vi "host.vi"() -> ()   [LabVIEW 2018]
uses:
  <vilib>/userdefined/High Color/nirio_resource_hc.ctl
  <instrlib>/niDCPower/nidcpower.llb/niDCPower Measurement Type.ctl
  <vilib>/FPGAPlugInAG/PXI-7953R/niLvFpga_Open_PXI-7953R.vi
  <vilib>/rvi/interface/common/dynamic/niFpgaDynamicAddResources.vi
  <vilib>/FPGAPlugInAG/Dynamic/niLvFpga_Reset_Dynamic.vi
  <vilib>/FPGAPlugInAG/Dynamic/niLvFpga_Run_Dynamic.vi
  <vilib>/Utility/error.llb/Error Cluster From Error Code.vi
  <vilib>/rvi/errors/niLvFpgaAdjustHostInterfaceError.vi
  <vilib>/FPGAPlugInAG/Dynamic/niLvFpga_Close_Dynamic.vi
  <vilib>/rvi/interface/nirviOpenFPGA/nirviOpenFPGA.xnode
  FPGA Bitfiles/matrix_FPGATarget_Matrixtarget_8M6uhoGy8lc.lvbitx
  <vilib>/rvi/interface/nirviMethod/nirviMethod.xnode
  <vilib>/rvi/interface/nirviReadWriteControl/nirviReadWriteControl.xnode
  <vilib>/rvi/interface/nirviCloseFPGA/nirviCloseFPGA.xnode
  <vilib>/FPGAPlugInAG/Dynamic/niLvFpga_ReadFifo_Dynamic.vi
  <vilib>/rvi/errors/niLvFpgaMergeErrorWithErrorCode.vi
  <vilib>/rvi/interface/Simulation/niFpgaSimulationCallBeginRW.vi
  <vilib>/vision/NI_Vision_Development_Module.lvlib
  NiFpgaLv.dll
panel:
  out "glitch_sum":i32=137
  in  "INIT_REGISTERS":bool
  out "Glitch Report":string="--Report-- 1\r\np0#R9 rd 29F  df  00219 \r\n--Report-- 1\r\np0#R9 rd 29F  df  00219 \r\n--Report-- 0\r\n\r\n--Report-- 0\r\n\r\n--Report-- 1\r\np1#R146 rd FF  df  BF1E \r\n--Report-- 0\r\n\r\n--Report-- 0\r\n\r\n--Report-- 0\r\n\r\n--Report-- 0\r\n\r\n--Report-- 0\r\n\r\n--Report-- 3\r\np0#R4 rd 1E7  df  00500 p0#R9 rd 432  df  00219 p1#R58 rd 300  df  200 \r\n--Report-- 3\r\np0#R4 rd 1E7  df  00500 p0#R9 rd 432  df  00219 p1#R58 rd 300  df  200 \r\n--Report-- 3\r\np0#R4 rd 1E7  df  00500 p0#R9 rd 432  df  00219 p1#R58 rd 300  df  200 \r\n--Report-- 3\r\np0#R4 rd 1E7  df  00500 p0#R9 rd 432  df  00219 p1#R58 rd 300  df  200 \r\n--Report-- 3\r\np0#R4 rd 1E7  df  00500 p0#R9 rd 432  df  00219 p1#R58 rd 300  df  200 \r\n--Report-- 0\r\n\r\n--Report-- 1\r\np0#R9 rd 29F  df  00219 \r\n--Report-- 0\r\n\r\n--Report-- 137\r\np1#R155 rd 3  df  200 p1#R157 rd 3  df  24AE p1#R159 rd 3  df  0 p1#R160 rd 3  df  500 p1#R161 rd 3  df  500 p1#R162 rd 3  df  0 p1#R163 rd 3  df  400 p1#R164 rd 3  df  400 p1#R165 rd 3  df  0 p1#R166 rd 3  df  500 p1#R167 rd 3  df  280 p1#R168 rd 3  df  0 p1#R169 rd 3  df  400 p1#R170 rd 3  df  200 p1#R174 rd 3  df  504 p1#R175 rd 3  df  10 p1#R179 rd 3  df  2 p1#R180 rd 3  df  20 p1#R181 rd 3  df  101 p1#R182 rd 3  df  110B p1#R183 rd 3  df  3C27 p1#R184 rd 3  df  110A p1#R185 rd 3  df  3222 p1#R186 rd 3  df  160B p1#R187 rd 3  df  3224 p2#R2 rd 3  df  6E p2#R3 rd 3  df  2923 p2#R4 rd 3  df  524 p2#R9 rd 3  df  92 p2#R10 rd 3  df  16 p2#R11 rd 3  df  8 p2#R12 rd 3  df  AB p2#R13 rd 3  df  93 p2#R14 rd 3  df  58 p2#R15 rd 3  df  4D p2#R16 rd 3  df  A9 p2#R17 rd 3  df  A0 p2#R21 rd 3  df  175 p2#R22 rd 3  df  16 p2#R23 rd 3  df  43 p2#R24 rd 3  df  C p2#R25 rd 3  df  0 p2#R26 rd 3  df  15 p2#R27 rd 3  df  1F p2#R28 rd 3  df  16 p2#R29 rd 3  df  98 p2#R30 rd 3  df  4C p2#R31 rd 3  df  A0 p2#R32 rd 3  df  C814 p2#R33 rd 3  df  8080 p2#R34 rd 3  df  D960 p2#R35 rd 3  df  D960 p2#R36 rd 3  df  7F00 p2#R38 rd 3  df  8000 p2#R39 rd 3  df  8008 p2#R40 rd 3  df  EF04 p2#R41 rd 3  df  8D73 p2#R42 rd 3  df  D0 p2#R43 rd 3  df  6020 p2#R44 rd 3  df  6020 p2#R45 rd 3  df  F0A0 p2#R46 rd 3  df  C4A p2#R47 rd 3  df  DF20 p2#R51 rd 3  df  146E p2#R54 rd 3  df  7810 p2#R55 rd 3  df  300 p2#R56 rd 3  df  440 p2#R57 rd 3  df  68C p2#R58 rd 3  df  68C p2#R59 rd 3  df  68C p2#R60 rd 3  df  68C p2#R61 rd 3  df  17D9 p2#R62 rd 3  df  1CFF p2#R70 rd 3  df  D900 p2#R87 rd 3  df  219 p2#R88 rd 3  df  284 p2#R89 rd 3  df  219 p2#R90 rd 3  df  284 p2#R92 rd 3  df  120C p2#R93 rd 3  df  1512 p2#R94 rd 3  df  683C p2#R95 rd 3  df  3008 p2#R96 rd 3  df  2 p2#R100 rd 3  df  59FC p2#R101 rd 3  df  0 p2#R103 rd 3  df  4010 p2#R104 rd 3  df  11 p2#R130 rd 3  df  3FC p2#R131 rd 3  df  301 p2#R132 rd 3  df  C1 p2#R133 rd 3  df  3A1 p2#R134 rd 3  df  3D4 p2#R135 rd 3  df  3D7 p2#R136 rd 3  df  399 p2#R137 rd 3  df  3F8 p2#R138 rd 3  df  1C p2#R139 rd 3  df  3BD p2#R140 rd 3  df  3DB p2#R141 rd 3  df  3BD p2#R142 rd 3  df  3FC p2#R143 rd 3  df  3DE p2#R144 rd 3  df  3DE p2#R145 rd 3  df  3DE p2#R146 rd 3  df  3DE p2#R147 rd 3  df  1F p2#R148 rd 3  df  41 p2#R149 rd 3  df  363 p2#R150 rd 3  df  0 p2#R152 rd 3  df  FF p2#R153 rd 3  df  1 p2#R156 rd 3  df  DF20 p2#R180 rd 3  df  20 p2#R198 rd 3  df  0 p2#R200 rd 3  df  0 p2#R203 rd 3  df  0 p2#R204 rd 3  df  0 p2#R205 rd 3  df  21A0 p2#R206 rd 3  df  1E9B p2#R207 rd 3  df  4A4A p2#R208 rd 3  df  168D p2#R209 rd 3  df  4D p2#R210 rd 3  df  0 p2#R211 rd 3  df  0 p2#R212 rd 3  df  208 p2#R213 rd 3  df  0 p2#R239 rd 3  df  8 p2#R242 rd 3  df  0 p2#R244 rd 3  df  6E p2#R246 rd 3  df  36 p2#R247 rd 3  df  D p2#R248 rd 3  df  AB p2#R249 rd 3  df  88 p2#R250 rd 3  df  48 p2#R251 rd 3  df  57 p2#R252 rd 3  df  5E p2#R253 rd 3  df  7A p2#R254 rd 3  df  503F \r\n"
  in  "REGISTERS":bool=TRUE
  in  "GLITCH":path=path "C:/TIM/Project/Matrix/Logs/Control/GLITCH"
  out "GLITCH_log file":refnum<file>
  in  "Index - Registers Page 2":u16[](array[numeric])=[2, 3, 4, 9, 10, 11, 12, 13, 14, 15, 16, 17, 65535, 65535, 65535, 21, 22, 23, 24, 25, 26, 27, 28, 29, 30, 31, 32, 33, 34, 35, 36, 38, 39, 40, 41, 42, 43, 44, 45, 46, 47, 65535, 65535, 65535, 51, 54, 55, 56, 57, 58, 59, 60, 61, 62, 65535, 70, 65535, 65535, 65535, 65535, 87, 88, 89, 90, 65535, 92, 93, 94, 95, 96, 65535, 65535, 65535, 100, 101, 103, 104, 130, 131, 132, 133, 134, 135, 136, 137, 138, 139, 140, 141, 142, 143, 144, 145, 146, 147, 148, 149, 150, 152, 153, 156, 180, 198, 200, 203, 204, 205, 206, 207, 208, 209, 210, 211, 212, 213, 239, 65535, 242, 65535, 244, 246, 247, 248, 249, 250, 251, 252, 253, 254, 255, 65535, 65535, 65535, 65535, 65535, 65535, 65535, 65535, 65534, 65535, 65535, 65531, 241, 242, 243, 244, 245, 246, 247, 248, 249, 250, 251, 252, 253, 254, 255]
  in  "Registers Page 2":u16[](array[numeric])=[110, 10531, 1316, 146, 22, 8, 171, 147, 88, 77, 169, 160, 65535, 65535, 65535, 373, 22, 67, 12, 0, 21, 31, 22, 152, 76, 160, 51220, 32896, 55648, 55648, 32512, 32768, 32776, 61188, 36211, 208, 24608, 24608, 61600, 3146, 57120, 65535, 65535, 65535, 5230, 30736, 768, 1088, 1676, 1676, 1676, 1676, 6105, 7423, 65535, 55552, 0, 65535, 65535, 65535, 537, 644, 537, 644, 2, 4620, 5394, 26684, 12296, 2, 32896, 65535, 65535, 23036, 0, 16400, 17, 1020, 769, 193, 929, 980, 983, 921, 1016, 28, 957, 987, 957, 1020, 990, 990, 990, 990, 31, 65, 867, 0, 255, 1, 57120, 32, 0, 0, 0, 0, 8608, 7835, 19018, 5773, 77, 0, 0, 520, 0, 8, 0, 0, 0, 110, 54, 13, 171, 136, 72, 87, 94, 122, 20543, 43136] format="%x"
  in  "current limit VDDIO":dbl=0.1 format="%#_13g"
  in  "voltage level VDDIO":dbl=2.5 format="%#_13g"
  in  "57":i16=57
  in  "91":i16=91
  in  "Index - Registers Page 1":u16[](array[numeric])=[5, 6, 8, 16, 17, 18, 27, 28, 30, 37, 52, 53, 58, 59, 60, 71, 72, 76, 77, 78, 82, 83, 84, 85, 86, 87, 88, 104, 128, 129, 130, 131, 132, 133, 134, 135, 136, 137, 138, 139, 140, 141, 142, 143, 144, 145, 146, 147, 148, 149, 155, 157, 159, 160, 161, 162, 163, 164, 165, 166, 167, 168, 169, 170, 174, 175, 179, 180, 181, 182, 183, 184, 185, 186, 187, 188, 189, 190, 191, 192, 193, 194, 195, 196, 200, 220, 221, 222, 223, 224, 225, 226, 227, 240]
  in  "Registers Page 1":u16[](array[numeric])=[3, 28686, 128, 61437, 64831, 16367, 0, 0, 512, 5, 16, 61456, 512, 1066, 1024, 24, 0, 0, 0, 10, 0, 7700, 17966, 34666, 47008, 57548, 0, 17, 7, 56588, 62696, 1276, 57868, 63212, 764, 56588, 62696, 250, 34866, 56754, 63466, 2, 47646, 60627, 63473, 255, 48926, 61142, 63474, 3, 512, 9390, 0, 1280, 1280, 0, 1024, 1024, 0, 1280, 640, 0, 1024, 512, 1284, 16, 2, 32, 257, 4363, 15399, 4362, 12834, 5643, 12836, 9228, 24124, 127, 8200, 20023, 100, 8463, 19250, 100, 0, 7700, 17966, 34666, 47008, 57548, 0, 28672, 45091, 0] format="%x"
  out "Glitch Registers":string="p1#R155 rd 3  df  200 p1#R157 rd 3  df  24AE p1#R159 rd 3  df  0 p1#R160 rd 3  df  500 p1#R161 rd 3  df  500 p1#R162 rd 3  df  0 p1#R163 rd 3  df  400 p1#R164 rd 3  df  400 p1#R165 rd 3  df  0 p1#R166 rd 3  df  500 p1#R167 rd 3  df  280 p1#R168 rd 3  df  0 p1#R169 rd 3  df  400 p1#R170 rd 3  df  200 p1#R174 rd 3  df  504 p1#R175 rd 3  df  10 p1#R179 rd 3  df  2 p1#R180 rd 3  df  20 p1#R181 rd 3  df  101 p1#R182 rd 3  df  110B p1#R183 rd 3  df  3C27 p1#R184 rd 3  df  110A p1#R185 rd 3  df  3222 p1#R186 rd 3  df  160B p1#R187 rd 3  df  3224 p2#R2 rd 3  df  6E p2#R3 rd 3  df  2923 p2#R4 rd 3  df  524 p2#R9 rd 3  df  92 p2#R10 rd 3  df  16 p2#R11 rd 3  df  8 p2#R12 rd 3  df  AB p2#R13 rd 3  df  93 p2#R14 rd 3  df  58 p2#R15 rd 3  df  4D p2#R16 rd 3  df  A9 p2#R17 rd 3  df  A0 p2#R21 rd 3  df  175 p2#R22 rd 3  df  16 p2#R23 rd 3  df  43 p2#R24 rd 3  df  C p2#R25 rd 3  df  0 p2#R26 rd 3  df  15 p2#R27 rd 3  df  1F p2#R28 rd 3  df  16 p2#R29 rd 3  df  98 p2#R30 rd 3  df  4C p2#R31 rd 3  df  A0 p2#R32 rd 3  df  C814 p2#R33 rd 3  df  8080 p2#R34 rd 3  df  D960 p2#R35 rd 3  df  D960 p2#R36 rd 3  df  7F00 p2#R38 rd 3  df  8000 p2#R39 rd 3  df  8008 p2#R40 rd 3  df  EF04 p2#R41 rd 3  df  8D73 p2#R42 rd 3  df  D0 p2#R43 rd 3  df  6020 p2#R44 rd 3  df  6020 p2#R45 rd 3  df  F0A0 p2#R46 rd 3  df  C4A p2#R47 rd 3  df  DF20 p2#R51 rd 3  df  146E p2#R54 rd 3  df  7810 p2#R55 rd 3  df  300 p2#R56 rd 3  df  440 p2#R57 rd 3  df  68C p2#R58 rd 3  df  68C p2#R59 rd 3  df  68C p2#R60 rd 3  df  68C p2#R61 rd 3  df  17D9 p2#R62 rd 3  df  1CFF p2#R70 rd 3  df  D900 p2#R87 rd 3  df  219 p2#R88 rd 3  df  284 p2#R89 rd 3  df  219 p2#R90 rd 3  df  284 p2#R92 rd 3  df  120C p2#R93 rd 3  df  1512 p2#R94 rd 3  df  683C p2#R95 rd 3  df  3008 p2#R96 rd 3  df  2 p2#R100 rd 3  df  59FC p2#R101 rd 3  df  0 p2#R103 rd 3  df  4010 p2#R104 rd 3  df  11 p2#R130 rd 3  df  3FC p2#R131 rd 3  df  301 p2#R132 rd 3  df  C1 p2#R133 rd 3  df  3A1 p2#R134 rd 3  df  3D4 p2#R135 rd 3  df  3D7 p2#R136 rd 3  df  399 p2#R137 rd 3  df  3F8 p2#R138 rd 3  df  1C p2#R139 rd 3  df  3BD p2#R140 rd 3  df  3DB p2#R141 rd 3  df  3BD p2#R142 rd 3  df  3FC p2#R143 rd 3  df  3DE p2#R144 rd 3  df  3DE p2#R145 rd 3  df  3DE p2#R146 rd 3  df  3DE p2#R147 rd 3  df  1F p2#R148 rd 3  df  41 p2#R149 rd 3  df  363 p2#R150 rd 3  df  0 p2#R152 rd 3  df  FF p2#R153 rd 3  df  1 p2#R156 rd 3  df  DF20 p2#R180 rd 3  df  20 p2#R198 rd 3  df  0 p2#R200 rd 3  df  0 p2#R203 rd 3  df  0 p2#R204 rd 3  df  0 p2#R205 rd 3  df  21A0 p2#R206 rd 3  df  1E9B p2#R207 rd 3  df  4A4A p2#R208 rd 3  df  168D p2#R209 rd 3  df  4D p2#R210 rd 3  df  0 p2#R211 rd 3  df  0 p2#R212 rd 3  df  208 p2#R213 rd 3  df  0 p2#R239 rd 3  df  8 p2#R242 rd 3  df  0 p2#R244 rd 3  df  6E p2#R246 rd 3  df  36 p2#R247 rd 3  df  D p2#R248 rd 3  df  AB p2#R249 rd 3  df  88 p2#R250 rd 3  df  48 p2#R251 rd 3  df  57 p2#R252 rd 3  df  5E p2#R253 rd 3  df  7A p2#R254 rd 3  df  503F "
  out "glitch_num":i32=137
  out "Data_Read":u16=3 format="%x"
  in  "Index - Registers Page 0":u16[](array[numeric])=[0, 1, 2, 3, 4, 5, 6, 7, 8, 9, 10, 11, 12, 13, 31, 32, 33, 34, 35, 36, 65535, 65535, 65535, 65535, 65535, 48, 49, 50, 51, 52, 54, 55, 65535, 60, 61, 65535, 63, 64, 65, 66, 89, 90, 95, 96, 65535, 65535, 65535, 65535, 101, 112, 113, 114, 115, 116, 117, 118, 119, 120, 121, 122, 123, 124, 125, 126, 128, 129, 130, 131, 132, 133, 134, 135, 200, 240, 245, 246, 247, 248, 65535, 250, 251, 252, 253, 255, 65535]
  in  "Registers Page 0":u16[](array[numeric])=[5178, 12, 30, 1024, 1280, 388, 42, 190, 17, 537, 17, 0, 0, 8, 0, 768, 1036, 297, 1544, 32875, 32, 32, 32, 32, 32, 1066, 7168, 0, 841, 49177, 61680, 0, 33, 6688, 8222, 8224, 8224, 8220, 215, 1911, 12, 49167, 8989, 128, 0, 0, 0, 0, 0, 31498, 31498, 6414, 6159, 22322, 22068, 29493, 12306, 30978, 29958, 30474, 30729, 32006, 12560, 126, 127, 127, 22282, 22539, 18188, 18446, 23298, 92, 0, 0, 2047, 2047, 0, 0, 124, 0, 0, 0, 0, 5178] format="%x"
  out "number":u64=515396075521 format="%b"
  in  "WRITE\nSEL_LOG":bool=TRUE caption="SEL LOGS"
  out "SEL_log file":refnum<file>
  out "IS_SEL":bool
  in  "SIM_SEL":bool
  in  "VDDIO_limit, mA":dbl=20.0 format="%#_13g"
  in  "VAA_limit, mA":dbl=40.0 format="%#_13g"
  out "selNumVAA":i32 caption="selNum"
  out "selNumVDDIO":i32 caption="selNum"
  in  "voltage level VAA":dbl=2.8 format="%#_13g"
  in  "voltage level VDD":dbl=2.8 format="%#_13g"
  in  "current limit VAA":dbl=0.10000000000000009 format="%#_13g"
  in  "current limit VDD":dbl=0.1 format="%#_13g"
  in  "SEL":path=path "C:/TIM/Project/Matrix/Logs/Control/SEL"
  out "Температура":string="0"
  out "Номер образца":string="0"
  out "VDDIO_Current, mA":dbl=-0.05343834220867134 caption="mA" format="%_2g"
  out "VDDIO_Voltage, V":dbl=2.500600525204199 caption="V" format="%_3g"
  out "VAA_Current, mA":dbl=14.9087718833614 caption="mA" format="%_2g"
  out "VAA_Voltage, V":dbl=2.800387385516999 caption="V" format="%_3g"
  in  "VAA - VAAPIX":refnum<k15>="PXI1Slot2"
  in  "SEL_time":u32=100
  out "Read_Low":u8=3 format="%x"
  out "Read_Up":u8 format="%x"
  out "TIRISTOR":bool
  in  "/RESET":bool=TRUE
  in  "DataLow":u8=25 format="%x"
  in  "Reg":u8=254 format="%x"
  in  "DataUp":u8=2 format="%x"
  in  "Device":u8=186 format="%x"
  in  "VDD_limit, mA":dbl=20.0 format="%#_13g"
  out "selNumVDD":i32 caption="selNum"
  out "Ready":bool=TRUE
  in  "output enabled":bool=TRUE
  out "VDD_Current, mA":dbl=-0.3667932165298103 caption="mA" format="%_2g"
  out "VDD_Voltage, V":dbl=2.7994963728933535 caption="V" format="%_3g"
  in  "VDDIO - VDD":refnum<k15>="PXI1Slot3"
  in  "Comand":T1(ring)
  in  "Height_pix":i32=250
  in  "Width_pix":i32=250
  in  "55":i16=55
  in  "73":i16=73
  in  "75":i16=75
  in  "56":i16=56
  in  "55":i16=55
  in  "Comand":bool
  out "ACK":u8 format="%b"
  out "String_counter":i16=250
  in  "String_number":i16=250
  in  "I2C_Request":bool
  in  "FALSE_LV":bool
  in  "FALSE_PIXCLK":bool=TRUE
  in  "TRUE_FV":bool=TRUE
  in  "1_EXTCLK_divider":i16=1
  out "Image":T2(plugin-control)
  in  "0_WE divider":i32
  in  "50_Rise/Fall divider":i32=25
  in  "72":i16=72
  in  "18":i16=18
  in  "36":i16=36
  in  "54":i16=54
  in  "71":i16=71
  in  "17":i16=17
  in  "35":i16=35
  in  "53":i16=53
  in  "75_Stop":i16=75
  in  "100_Sclk_divider":i32=50
  in  "Read1":u8=255 format="%x"
  in  "Read2":u8=255 format="%x"
  in  "I2C_Write":bool
  in  "stop":bool=TRUE
  out "ArrayUp":u64=1432
  out "ArrayLow":u64=27021700977551334
  in  "resource name":T3="PXI1Slot6" caption="RIO Device"
  out "Сколько вначале":u32=262142
  out "Data":u8[](array[numeric])
  # "YCbCr mode"
  # "RGB565"
  # "VDD"
  # "VDDIO"
  # "VAA"
  # "I2C"
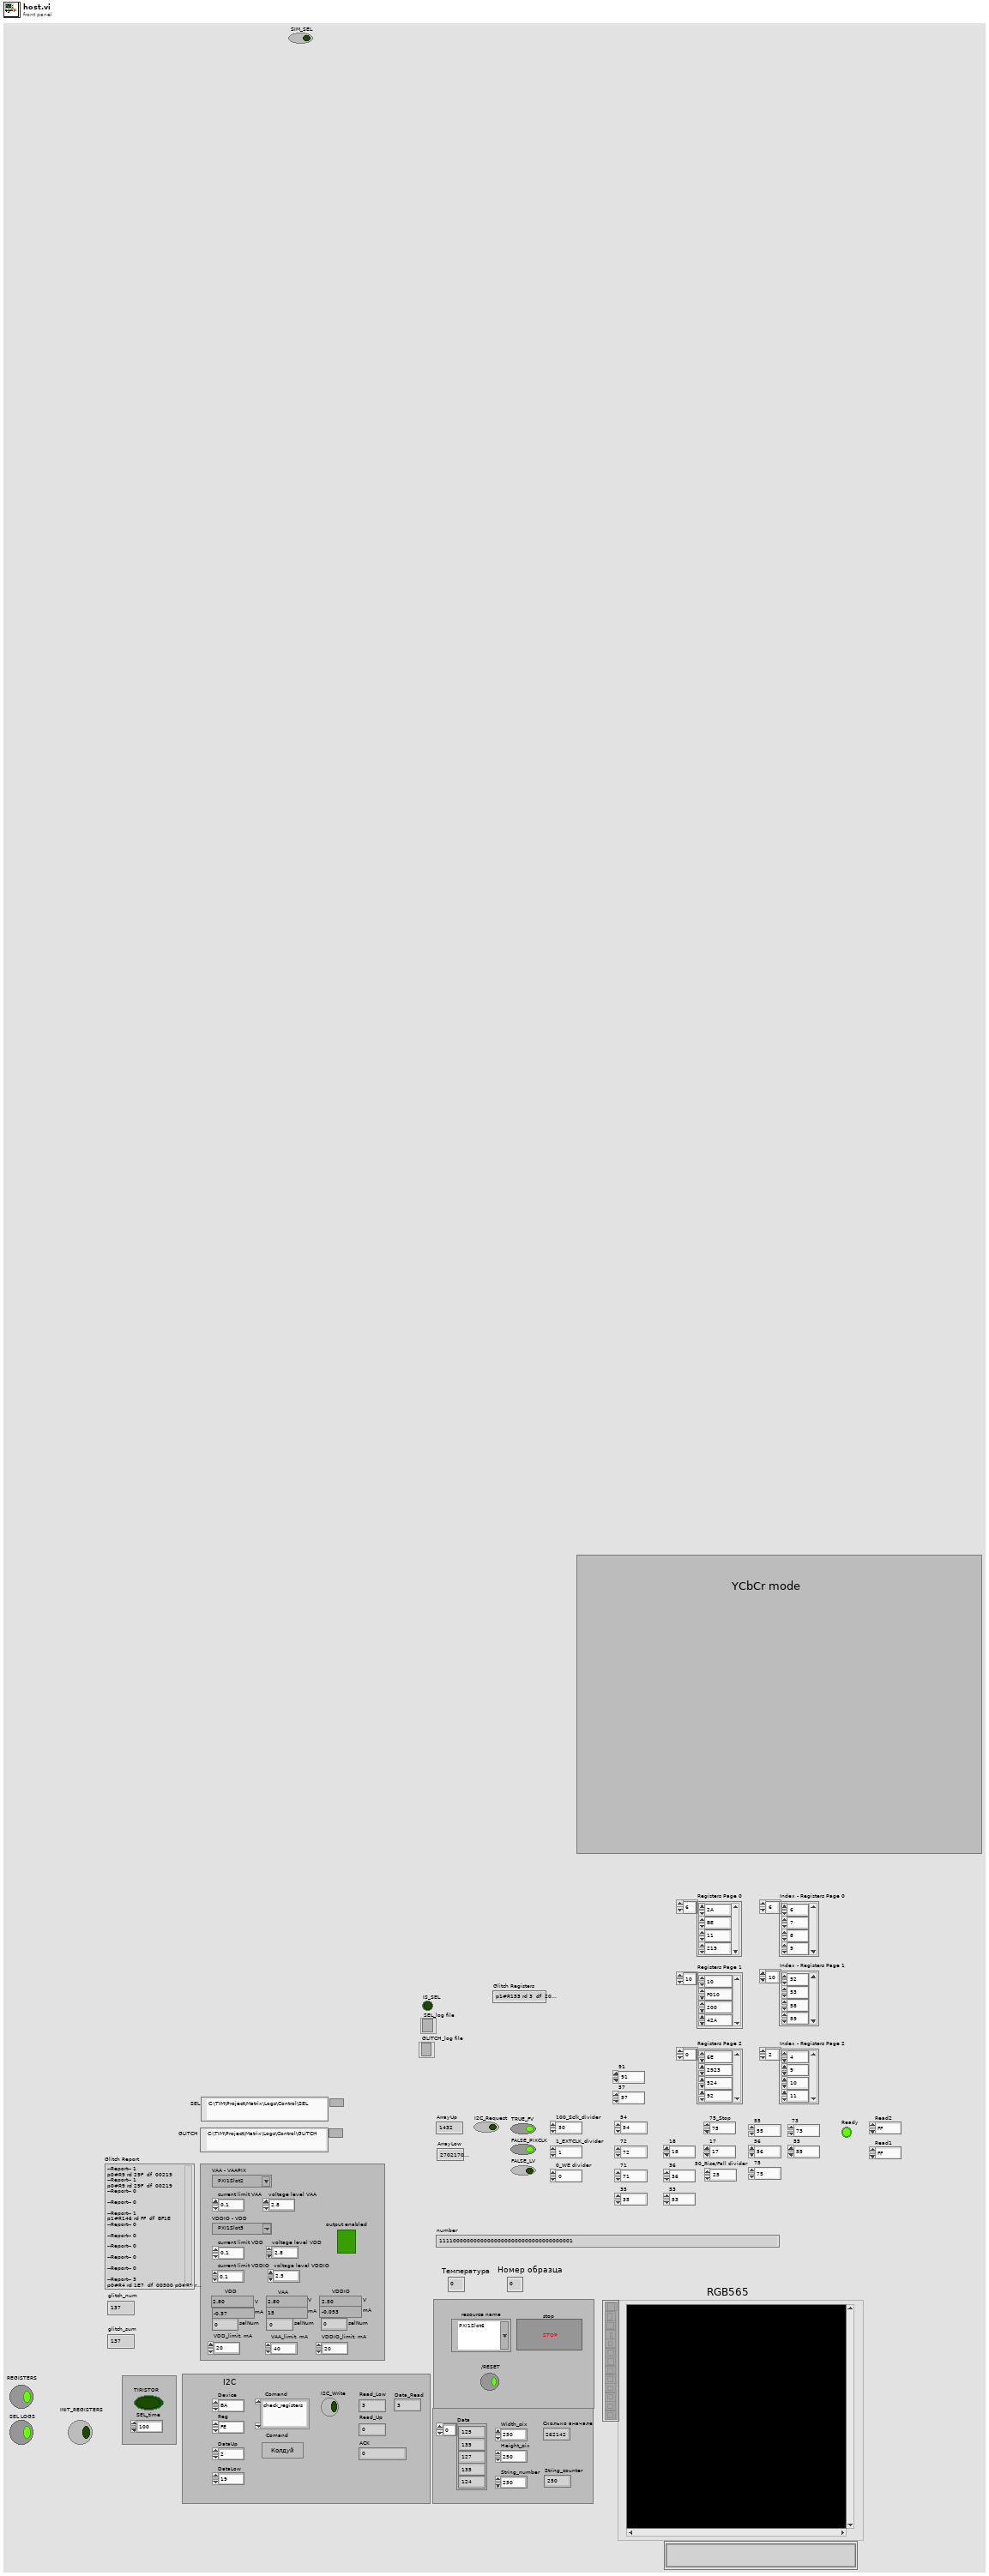
[diagram p1: front panel]
types:
  T1 = enum16{"check_registers", "From Controls", "250x250", "RGB565"}
  T2 = typedef "IMAQ Image.ctl" = refnum<image>
  T3 = typedef "nirio_resource_hc.ctl" = tag
  T4 = enum16{"open", "replace", "create", "open or create", "replace or create", "replace or create with confirmation"}
  T5 = typedef "niDCPower Measurement Type.ctl" = i32
  T6 = typedef "Image Type" = u32
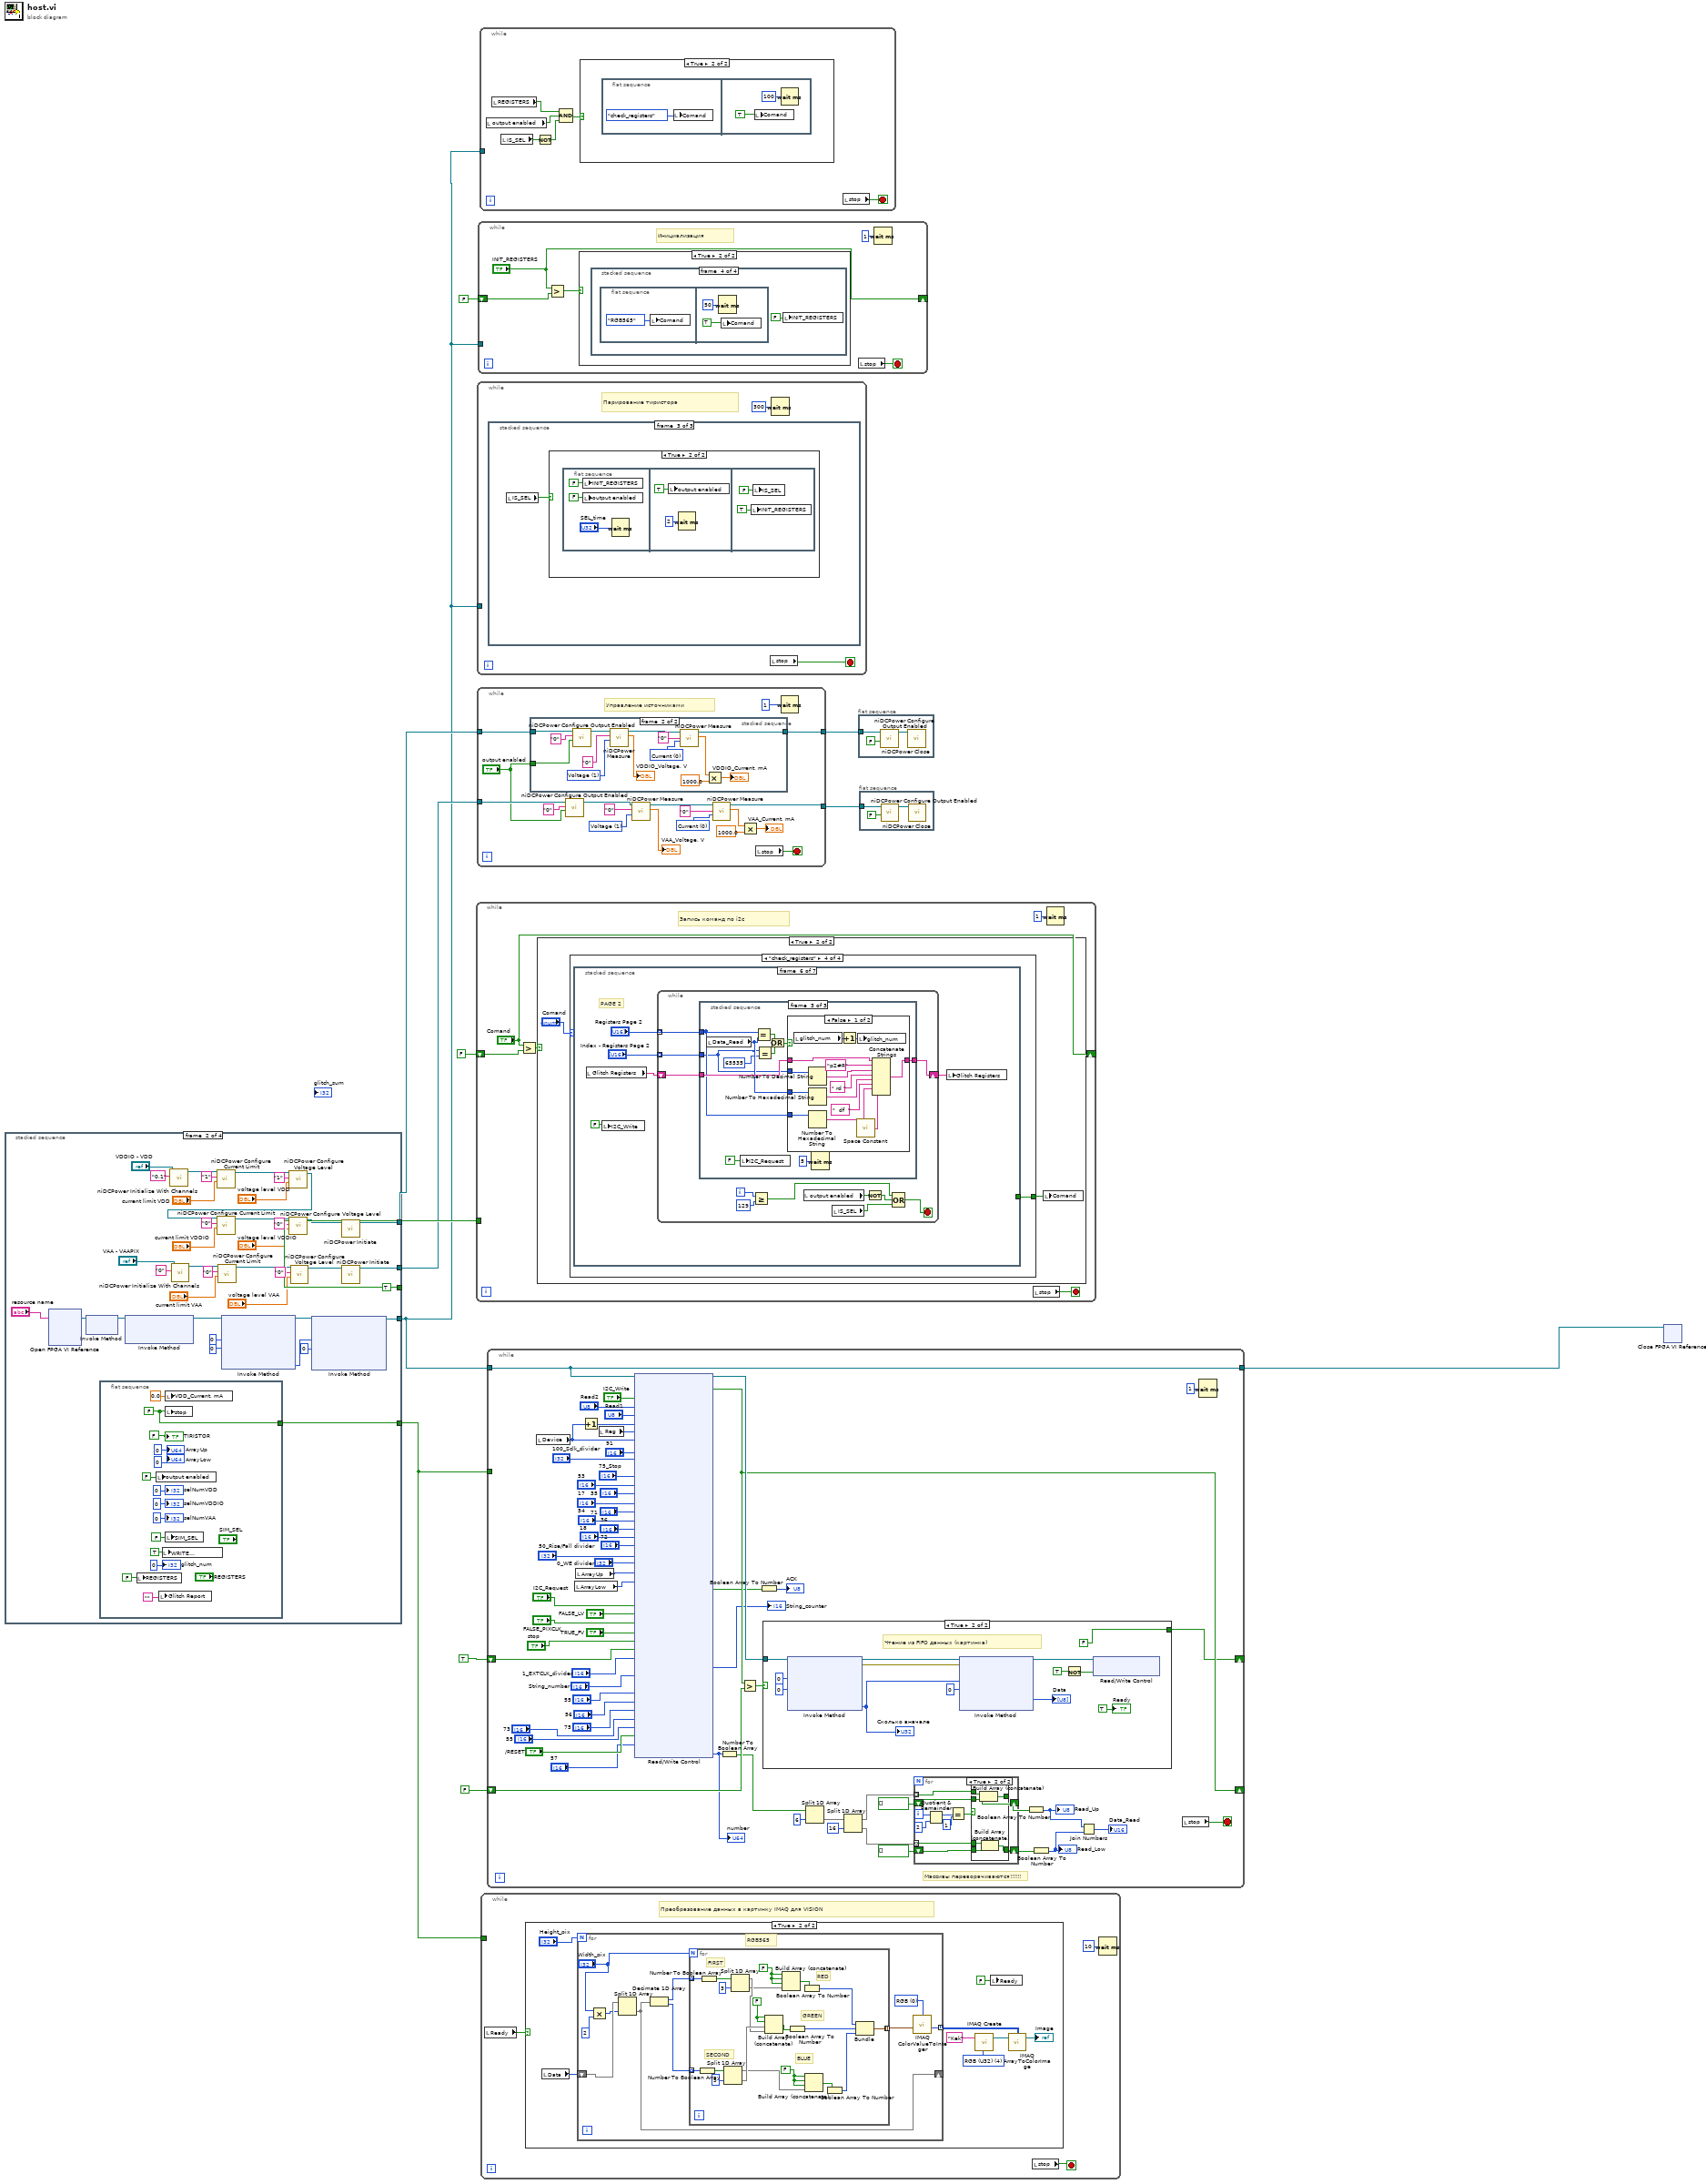
[diagram p0: block diagram]
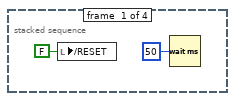
[diagram p3: hidden frame]
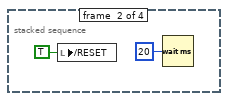
[diagram p4: hidden frame]
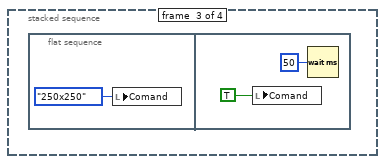
[diagram p5: hidden frame]
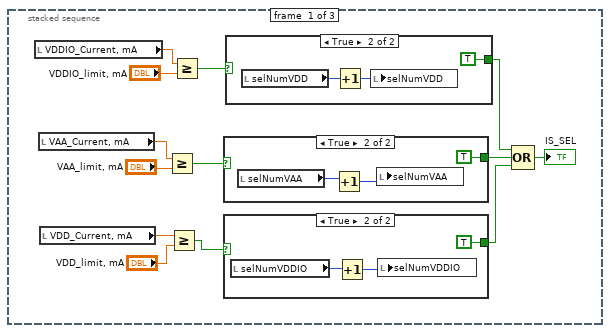
[diagram p8: hidden frame]
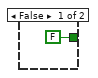
[diagram p9: hidden frame]
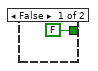
[diagram p10: hidden frame]
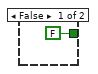
[diagram p11: hidden frame]
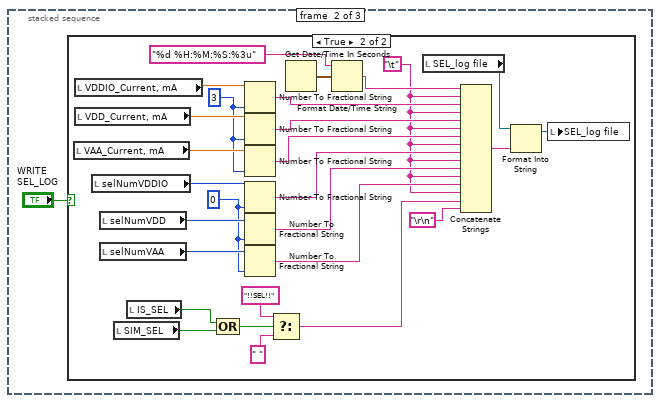
[diagram p12: hidden frame]
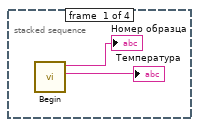
[diagram p15: hidden frame]
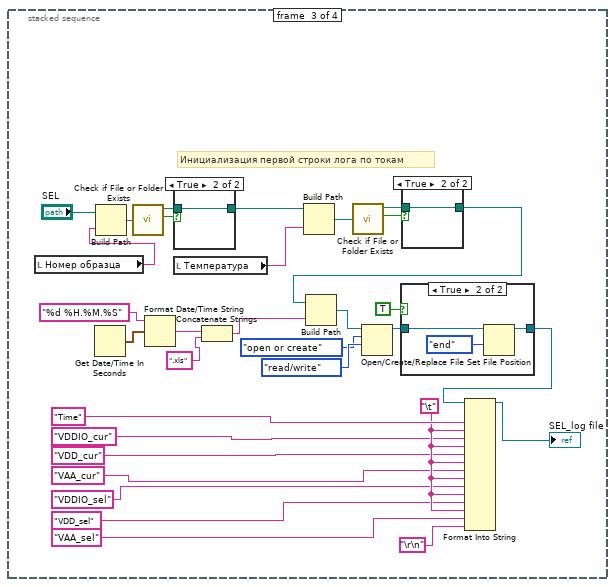
[diagram p16: hidden frame]
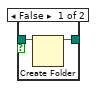
[diagram p18: hidden frame]
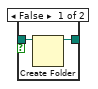
[diagram p19: hidden frame]
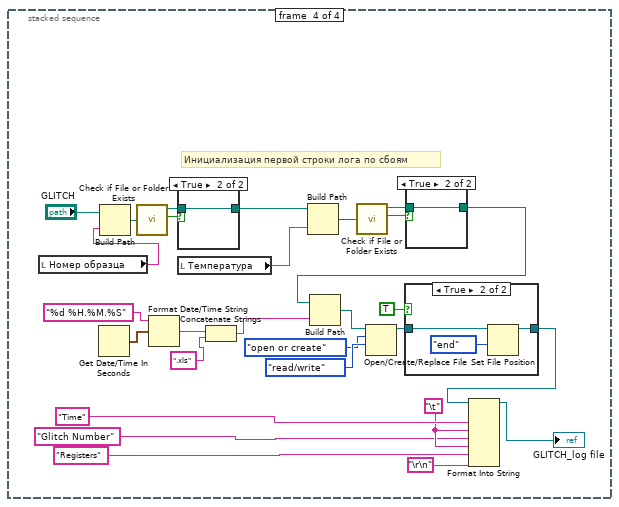
[diagram p20: hidden frame]
diagram:
  n1 = stacked-sequence {
    tunnel: [_ w52 _ _] -> w2
    tunnel: [_ w34 _ _] -> w5
    tunnel: [_ w33 _ _] -> w7
    tunnel: [_ TRUE _ _] -> w6
    tunnel: [_ w22 _ _] -> w4
    frame #0 {
      n2 = call "Begin.vi"() -> ("Температура 2"=→"Температура":string, "Номер образца 2"=→"Номер образца":string)  [unwired: 10 in]
    }
    frame #1 {
      n3 = xnode "Open FPGA VI Reference"("resource name"="resource name") -> ("FPGA VI Reference Out"=w43:refnum<k20>)  [unwired: 1 in, 1 out]
      n4 = xnode "Invoke Method"("FPGA VI Reference In"=w43) -> ("FPGA VI Reference Out"=w42:refnum<k20>)  [unwired: 1 in, 1 out]
      n5 = flat-sequence {
        tunnel: [w66] -> w34
        frame #0 {
          w66 = FALSE ("СТОП ПЛИС")
          n6 = local write "REGISTERS"(FALSE ("REGISTERS")) -> ()
          n7 = local write "output enabled"(FALSE ("output enabled")) -> ()
          n8 = local write "Glitch Report"("") -> ()
          n9 = local write "WRITE\nSEL_LOG"(TRUE ("WRITE\nSEL_LOG")) -> ()
          n10 = local write "VDD_Current, mA"(0.0 ("Ch1_Current, mA")) -> ()
          n11 = local write "stop"(w66) -> ()
          n12 = local write "SIM_SEL"(FALSE ("SIM_SEL")) -> ()
          "ArrayLow" <- u64 0 ("ArrayLow")
          "ArrayUp" <- u64 0 ("ArrayUp")
          "selNumVDD" <- 0 ("Numeric")
          "TIRISTOR" <- FALSE ("TIRISTOR")
          "selNumVDDIO" <- 0 ("Numeric")
          "selNumVAA" <- 0 ("Numeric")
          "glitch_num" <- 0 ("glitch_num")
        }
      }
      n13 = xnode "Invoke Method"("FPGA VI Reference In"=w42) -> ("FPGA VI Reference Out"=w40:refnum<k20>)  [unwired: 2 in, 1 out]
      n14 = call <instrlib>:"niDCPower Initialize With Channels.vi"("channels"="0,1", "resource name"="VDDIO - VDD") -> ("instrument handle out"=w44:refnum<k15>)  [unwired: 8 in, 1 out]
      n15 = call <instrlib>:"niDCPower Initialize With Channels.vi"("channels"="0", "resource name"="VAA - VAAPIX") -> ("instrument handle out"=w23:refnum<k15>)  [unwired: 8 in, 1 out]
      n16 = call <instrlib>:"niDCPower Configure Current Limit.vi"("current limit"="current limit VDD", "channel name"="1", "instrument handle"=w44) -> ("instrument handle out"=w45:refnum<k15>)  [unwired: 7 in, 1 out]
      n17 = call <instrlib>:"niDCPower Configure Current Limit.vi"("current limit"="current limit VAA", "channel name"="0", "instrument handle"=w23) -> ("instrument handle out"=w24:refnum<k15>)  [unwired: 7 in, 1 out]
      n18 = xnode "Invoke Method"("FPGA VI Reference In"=w40, "Number of Elements"=u32 0, "Timeout (ms)"=0) -> ("FPGA VI Reference Out"=w38:refnum<k20>, "Elements Remaining"=w39:u32)  [unwired: 1 in, 2 out]
      n19 = call <instrlib>:"niDCPower Configure Voltage Level.vi"("voltage level"="voltage level VDD", "channel name"="1", "instrument handle"=w45) -> ("instrument handle out"=w15:refnum<k15>)  [unwired: 7 in, 1 out]
      n20 = call <instrlib>:"niDCPower Configure Current Limit.vi"("current limit"="current limit VDDIO", "channel name"="0", "instrument handle"=w15) -> ("instrument handle out"=w21:refnum<k15>)  [unwired: 7 in, 1 out]
      n21 = call <instrlib>:"niDCPower Configure Voltage Level.vi"("voltage level"="voltage level VDDIO", "channel name"="0", "instrument handle"=w21) -> ("instrument handle out"=w16:refnum<k15>)  [unwired: 7 in, 1 out]
      n22 = call <instrlib>:"niDCPower Configure Voltage Level.vi"("voltage level"="voltage level VAA", "channel name"="0", "instrument handle"=w24) -> ("instrument handle out"=w25:refnum<k15>)  [unwired: 7 in, 1 out]
      n23 = xnode "Invoke Method"("FPGA VI Reference In"=w38, "Number of Elements"=w39, "Timeout (ms)"=0) -> ("FPGA VI Reference Out"=w52:refnum<k20>)  [unwired: 1 in, 3 out]
      n24 = call <instrlib>:"niDCPower Initiate.vi"("instrument handle"=w16) -> ("instrument handle out"=w33:refnum<k15>)  [unwired: 9 in, 1 out]
      n25 = call <instrlib>:"niDCPower Initiate.vi"("instrument handle"=w25) -> ("instrument handle out"=w22:refnum<k15>)  [unwired: 9 in, 1 out]
    }
    frame #2 {
      w75 = "\t"
      # "Инициализация первой строки лога по токам"
      n26 = local read "Номер образца"() -> (w86:string)
      n27 = Get Date/Time In Seconds() -> (seconds since 1Jan1904=w91:timestamp)
      n28 = Build Path(base path="SEL", name or relative path=w86) -> (appended path=w84:path)
      n29 = call <vilib>:"Check if File or Folder Exists.vi"("path"=w84) -> ("file or folder exists?"=w83:bool, "dup path"=w82:path)  [unwired: 8 in, 1 out]
      n30 = Format Date/Time String(time format string (%c)="%d %H.%M.%S", seconds (now)=w91) -> (date/time string=w93:string)  [unwired: 1 in]
      n31 = case shown="True" w83 {
        tunnel: w82 -> [w107 w108]
        tunnel: [w106 w108] -> w88
        frame False {
          n32 = Create Folder(path (use dialog)=w107) -> (created path=w106:path)  [unwired: 2 in, 2 out]
        }
        frame True {
        }
      }
      n33 = local read "Температура"() -> (w89:string)
      n34 = Concatenate Strings(w93, ".xls" ("string")) -> (w94:string)
      n35 = Build Path(base path=w88, name or relative path=w89) -> (appended path=w97:path)
      n36 = call <vilib>:"Check if File or Folder Exists.vi"("path"=w97) -> ("file or folder exists?"=w98:bool, "dup path"=w87:path)  [unwired: 8 in, 1 out]
      n37 = case shown="True" w98 {
        tunnel: w87 -> [w104 w105]
        tunnel: [w103 w105] -> w95
        frame False {
          n38 = Create Folder(path (use dialog)=w104) -> (created path=w103:path)  [unwired: 2 in, 2 out]
        }
        frame True {
        }
      }
      n39 = Build Path(base path=w95, name or relative path=w94) -> (appended path=w92:path)
      n40 = Open/Create/Replace File(file path (use dialog)=w92, operation (0:open)=T4."open or create", access (0:read/write)=enum16{"read/write", "read-only", "write-only"}."read/write") -> (refnum out=w90:refnum<file>)  [unwired: 3 in, 2 out]
      n41 = case shown="True" TRUE {
        tunnel: w90 -> [w99 w102]
        tunnel: [w99 w100] -> w96
        frame False {
        }
        frame True {
          n42 = Set File Position(refnum=w102, from (0:start)=enum16{"start", "end", "current"}."end") -> (refnum out=w100:refnum<file>)  [unwired: 2 in, 1 out]
        }
      }
      n43 = Format Into String(initial string=w96, "Time" ("input 1"), w75, "VDDIO_cur" ("input 1"), w75, "VDD_cur" ("input 1"), w75, "VAA_cur" ("input 1"), w75, "VDDIO_sel" ("input 1"), w75, "VDD_sel" ("input 1"), w75, "VAA_sel" ("input 1"), "\r\n") -> (resulting string=→"SEL_log file":refnum<file>)  [unwired: 2 in, 1 out]
    }
    frame #3 {
      w113 = "\t"
      # "Инициализация первой строки лога по сбоям"
      n44 = local read "Номер образца"() -> (w124:string)
      n45 = Get Date/Time In Seconds() -> (seconds since 1Jan1904=w129:timestamp)
      n46 = Build Path(base path="GLITCH", name or relative path=w124) -> (appended path=w122:path)
      n47 = call <vilib>:"Check if File or Folder Exists.vi"("path"=w122) -> ("file or folder exists?"=w121:bool, "dup path"=w120:path)  [unwired: 8 in, 1 out]
      n48 = Format Date/Time String(time format string (%c)="%d %H.%M.%S", seconds (now)=w129) -> (date/time string=w131:string)  [unwired: 1 in]
      n49 = case shown="True" w121 {
        tunnel: w120 -> [w145 w146]
        tunnel: [w144 w146] -> w126
        frame False {
          n50 = Create Folder(path (use dialog)=w145) -> (created path=w144:path)  [unwired: 2 in, 2 out]
        }
        frame True {
        }
      }
      n51 = local read "Температура"() -> (w127:string)
      n52 = Concatenate Strings(w131, ".xls" ("string")) -> (w132:string)
      n53 = Build Path(base path=w126, name or relative path=w127) -> (appended path=w135:path)
      n54 = call <vilib>:"Check if File or Folder Exists.vi"("path"=w135) -> ("file or folder exists?"=w136:bool, "dup path"=w125:path)  [unwired: 8 in, 1 out]
      n55 = case shown="True" w136 {
        tunnel: w125 -> [w142 w143]
        tunnel: [w141 w143] -> w133
        frame False {
          n56 = Create Folder(path (use dialog)=w142) -> (created path=w141:path)  [unwired: 2 in, 2 out]
        }
        frame True {
        }
      }
      n57 = Build Path(base path=w133, name or relative path=w132) -> (appended path=w130:path)
      n58 = Open/Create/Replace File(file path (use dialog)=w130, operation (0:open)=T4."open or create", access (0:read/write)=enum16{"read/write", "read-only", "write-only"}."read/write") -> (refnum out=w128:refnum<file>)  [unwired: 3 in, 2 out]
      n59 = case shown="True" TRUE {
        tunnel: w128 -> [w137 w140]
        tunnel: [w137 w138] -> w134
        frame False {
        }
        frame True {
          n60 = Set File Position(refnum=w140, from (0:start)=enum16{"start", "end", "current"}."end") -> (refnum out=w138:refnum<file>)  [unwired: 2 in, 1 out]
        }
      }
      n61 = Format Into String(initial string=w134, "Time" ("input 1"), w113, "Glitch Number" ("input 1"), w113, "Registers" ("input 1"), "\r\n") -> (resulting string=→"GLITCH_log file":refnum<file>)  [unwired: 2 in, 1 out]
    }
  }
  n62 = while {
    shift-right: ["Comand"] -> _
    shift-left: FALSE -> [w149]
    tunnel: w6 -> [_]
    stop <- w151 stop-if-true
    # "Запись команд по i2c"
    n63 = Greater?(x="Comand", y=w149) -> (0:w150:bool)
    n64 = case shown="True" w150 {
      frame False {
      }
      frame True {
        n65 = case shown="\"check_registers\"" "Comand" {
          tunnel: [w154 w180 w205 w217] -> w152
          frame "RGB565" {
            n66 = stacked-sequence {
              tunnel: [_ w166] -> w154
              frame #0 {
                n67 = flat-sequence {
                  frame #0 {
                    n68 = local write "I2C_Write"(TRUE ("I2C_Write")) -> ()
                    n69 = call "I2C_Write.vi"("DataLow"=u8 1 ("Device"), "DataUp"=u8 0 ("Device"), "Reg"=u8 240 ("Device"), "Device"=u8 186) -> ("ArrayLow"=w160:u64, "ArrayUp"=w159:u64)  [unwired: 6 in]
                    n70 = local write "ArrayUp"(w159) -> ()
                    n71 = local write "ArrayLow"(w160) -> ()
                  }
                  frame #1 {
                    n72 = local write "I2C_Request"(TRUE ("I2C_Request")) -> ()
                    n73 = Wait (ms)(milliseconds to wait=u32 5) -> ()  [unwired: 1 out]
                  }
                  frame #2 {
                    n74 = local write "I2C_Request"(FALSE ("I2C_Request")) -> ()
                    n75 = Wait (ms)(milliseconds to wait=u32 5) -> ()  [unwired: 1 out]
                  }
                }
              }
              frame #1 {
                n76 = flat-sequence {
                  tunnel: [FALSE ("RGB565")] -> w166
                  frame #0 {
                    n77 = local write "I2C_Write"(TRUE ("I2C_Write")) -> ()
                    n78 = call "I2C_Write.vi"("DataLow"=u8 0 ("Device"), "DataUp"=u8 3 ("Device"), "Reg"=u8 58 ("Device"), "Device"=u8 186) -> ("ArrayLow"=w172:u64, "ArrayUp"=w171:u64)  [unwired: 6 in]
                    n79 = local write "ArrayUp"(w171) -> ()
                    n80 = local write "ArrayLow"(w172) -> ()
                  }
                  frame #1 {
                    n81 = local write "I2C_Request"(TRUE ("I2C_Request")) -> ()
                    n82 = Wait (ms)(milliseconds to wait=u32 2) -> ()  [unwired: 1 out]
                  }
                  frame #2 {
                    n83 = local write "I2C_Request"(FALSE ("I2C_Request")) -> ()
                    n84 = Wait (ms)(milliseconds to wait=u32 2) -> ()  [unwired: 1 out]
                  }
                }
              }
            }
          }
          frame "250x250" {
            w179 = 250 ("Height_pix")
            n85 = stacked-sequence {
              tunnel: [_ w192] -> w180
              frame #0 {
                n86 = flat-sequence {
                  frame #0 {
                    n87 = local write "I2C_Write"(TRUE ("I2C_Write")) -> ()
                    n88 = call "I2C_Write.vi"("DataLow"=u8 0 ("Device"), "DataUp"=u8 0 ("Device"), "Reg"=u8 240 ("Device"), "Device"=u8 186) -> ("ArrayLow"=w186:u64, "ArrayUp"=w185:u64)  [unwired: 6 in]
                    n89 = local write "ArrayUp"(w185) -> ()
                    n90 = local write "ArrayLow"(w186) -> ()
                  }
                  frame #1 {
                    n91 = local write "I2C_Request"(TRUE ("I2C_Request")) -> ()
                    n92 = Wait (ms)(milliseconds to wait=u32 10) -> ()  [unwired: 1 out]
                  }
                  frame #2 {
                    n93 = local write "I2C_Request"(FALSE ("I2C_Request")) -> ()
                    n94 = Wait (ms)(milliseconds to wait=u32 10) -> ()  [unwired: 1 out]
                  }
                }
              }
              frame #1 {
                n95 = flat-sequence {
                  tunnel: [FALSE ("RGB565")] -> w192
                  frame #0 {
                    n96 = local write "I2C_Write"(TRUE ("I2C_Write")) -> ()
                    n97 = call "I2C_Write.vi"("DataLow"=u8 231 ("Device"), "DataUp"=u8 1 ("Device"), "Reg"=u8 4 ("Device"), "Device"=u8 186) -> ("ArrayLow"=w194:u64, "ArrayUp"=w193:u64)  [unwired: 6 in]
                    n98 = local write "ArrayUp"(w193) -> ()
                    n99 = local write "ArrayLow"(w194) -> ()
                  }
                  frame #1 {
                    n100 = local write "I2C_Request"(TRUE ("I2C_Request")) -> ()
                    n101 = Wait (ms)(milliseconds to wait=u32 10) -> ()  [unwired: 1 out]
                  }
                  frame #2 {
                    n102 = local write "I2C_Request"(FALSE ("I2C_Request")) -> ()
                    n103 = Wait (ms)(milliseconds to wait=u32 10) -> ()  [unwired: 1 out]
                  }
                }
              }
            }
            n104 = local write "String_number"(w179) -> ()
            n105 = local write "Width_pix"(w179) -> ()
            n106 = local write "Height_pix"(w179) -> ()
          }
          frame "From Controls" {
            n107 = flat-sequence {
              tunnel: [FALSE] -> w205
              frame #0 {
                n108 = call "I2C_Write.vi"("DataLow"="DataLow", "DataUp"="DataUp", "Reg"="Reg", "Device"="Device") -> ("ArrayLow"=w207:u64, "ArrayUp"=w206:u64)  [unwired: 6 in]
                n109 = local write "ArrayUp"(w206) -> ()
                n110 = local write "ArrayLow"(w207) -> ()
              }
              frame #1 {
                n111 = local write "I2C_Request"(TRUE ("I2C_Request")) -> ()
                n112 = Wait (ms)(milliseconds to wait=u32 5) -> ()  [unwired: 1 out]
              }
              frame #2 {
                n113 = local write "I2C_Request"(FALSE ("I2C_Request")) -> ()
                n114 = Wait (ms)(milliseconds to wait=u32 5) -> ()  [unwired: 1 out]
              }
            }
          }
          frame "check_registers" {
            n115 = stacked-sequence {
              tunnel: [_ _ _ _ _ _ FALSE ("RGB565")] -> w217
              frame #0 {
                n116 = flat-sequence {
                  frame #0 {
                    n117 = local write "I2C_Write"(TRUE ("I2C_Write")) -> ()
                    n118 = call "I2C_Write.vi"("DataLow"=u8 0 ("Device"), "DataUp"=u8 0 ("Device"), "Reg"=u8 240 ("Device"), "Device"=u8 186) -> ("ArrayLow"=w223:u64, "ArrayUp"=w222:u64)  [unwired: 6 in]
                    n119 = local write "ArrayUp"(w222) -> ()
                    n120 = local write "ArrayLow"(w223) -> ()
                  }
                  frame #1 {
                    n121 = local write "I2C_Request"(TRUE ("I2C_Request")) -> ()
                    n122 = Wait (ms)(milliseconds to wait=u32 5) -> ()  [unwired: 1 out]
                  }
                  frame #2 {
                    n123 = local write "I2C_Request"(FALSE ("I2C_Request")) -> ()
                    n124 = Wait (ms)(milliseconds to wait=u32 5) -> ()  [unwired: 1 out]
                  }
                }
              }
              frame #1 {
                # "PAGE 0"
                n125 = local write "glitch_num"(0 ("glitch_num")) -> ()
                n126 = local write "I2C_Write"(FALSE ("I2C_Write")) -> ()
                n127 = while {
                  tunnel: "Index - Registers Page 0" -> [w245] mode=indexing
                  tunnel: "Registers Page 0" -> [w244] mode=indexing
                  shift-right: [w242] -> w231
                  shift-left: "" -> [w243]
                  i -> [w238]
                  stop <- w236 stop-if-true
                  n128 = stacked-sequence {
                    tunnel: w245 -> [w247 _ w251]
                    tunnel: w244 -> [_ _ w256]
                    tunnel: w243 -> [_ _ w260]
                    tunnel: [_ _ w259] -> w242
                    frame #0 {
                      n129 = local write "Device"(u8 186 ("Device")) -> ()
                      n130 = local write "Reg"(w247) -> ()
                      n131 = Wait (ms)(milliseconds to wait=u32 1) -> ()  [unwired: 1 out]
                    }
                    frame #1 {
                      n132 = local write "I2C_Request"(TRUE ("I2C_Request")) -> ()
                      n133 = Wait (ms)(milliseconds to wait=u32 7) -> ()  [unwired: 1 out]
                    }
                    frame #2 {
                      n134 = local read "Data_Read"() -> (w258:u16)
                      n135 = local write "I2C_Request"(FALSE ("I2C_Request")) -> ()
                      n136 = Equal?(x=w256, y=w258) -> (x = y?=w253:bool)
                      n137 = Equal?(x=w251, y=u16 65535) -> (x = y?=w255:bool)
                      n138 = Or(x=w253, y=w255) -> (x .or. y?=w252:bool)
                      n139 = case shown="False" w252 {
                        tunnel: w260 -> [w273 w276]
                        tunnel: [w272 w276] -> w259
                        tunnel: w251 -> [w270 _]
                        tunnel: w258 -> [w266 _]
                        tunnel: w256 -> [w262 _]
                        frame False {
                          n140 = local read "glitch_num"() -> (w275:i32)
                          n141 = Number To Hexadecimal String(2:w262) -> (0:w264:string)  [unwired: 1 in]
                          n142 = Number To Hexadecimal String(2:w266) -> (0:w268:string)  [unwired: 1 in]
                          n143 = Number To Decimal String(number=w270) -> (decimal integer string=w269:string)  [unwired: 1 in]
                          n144 = Increment(x=w275) -> (x+1=w274:i32)
                          n145 = call <vilib>:"Space Constant.vi"() -> ("String"=w263:string)
                          n146 = local write "glitch_num"(w274) -> ()
                          n147 = Concatenate Strings(w273, "p0#R" ("string"), w269, " rd ", w268, "  df  ", w264, w263) -> (w272:string)
                        }
                        frame True {
                        }
                      }
                      n148 = Wait (ms)(milliseconds to wait=u32 5) -> ()  [unwired: 1 out]
                    }
                  }
                  n149 = Greater Or Equal?(x=w238, y=82) -> (x >= y?=w239:bool)
                  n150 = local read "output enabled"() -> (w241:bool)
                  n151 = local read "IS_SEL"() -> (w235:bool)
                  n152 = Not(x=w241) -> (.not. x?=w240:bool)
                  n153 = Compound Arithmetic op=OR(w239, w240, w235) -> (w236:bool)
                }
                "Glitch Registers" <- w231
              }
              frame #2 {
                n154 = flat-sequence {
                  frame #0 {
                    n155 = local write "I2C_Write"(TRUE ("I2C_Write")) -> ()
                    n156 = call "I2C_Write.vi"("DataLow"=u8 1 ("Device"), "DataUp"=u8 0 ("Device"), "Reg"=u8 240 ("Device"), "Device"=u8 186) -> ("ArrayLow"=w282:u64, "ArrayUp"=w281:u64)  [unwired: 6 in]
                    n157 = local write "ArrayUp"(w281) -> ()
                    n158 = local write "ArrayLow"(w282) -> ()
                  }
                  frame #1 {
                    n159 = local write "I2C_Request"(TRUE ("I2C_Request")) -> ()
                    n160 = Wait (ms)(milliseconds to wait=u32 5) -> ()  [unwired: 1 out]
                  }
                  frame #2 {
                    n161 = local write "I2C_Request"(FALSE ("I2C_Request")) -> ()
                    n162 = Wait (ms)(milliseconds to wait=u32 5) -> ()  [unwired: 1 out]
                  }
                }
              }
              frame #3 {
                # "PAGE 1"
                n163 = local read "Glitch Registers"() -> (w289:string)
                n164 = local write "I2C_Write"(FALSE ("I2C_Write")) -> ()
                n165 = while {
                  tunnel: "Index - Registers Page 1" -> [w300] mode=indexing
                  tunnel: "Registers Page 1" -> [w303] mode=indexing
                  shift-right: [w301] -> w288
                  shift-left: w289 -> [w302]
                  i -> [w294]
                  stop <- w296 stop-if-true
                  n166 = stacked-sequence {
                    tunnel: w300 -> [w305 _ w310]
                    tunnel: w303 -> [_ _ w314]
                    tunnel: w302 -> [_ _ w317]
                    tunnel: [_ _ w316] -> w301
                    frame #0 {
                      n167 = local write "Device"(u8 186 ("Device")) -> ()
                      n168 = local write "Reg"(w305) -> ()
                      n169 = Wait (ms)(milliseconds to wait=u32 1) -> ()  [unwired: 1 out]
                    }
                    frame #1 {
                      n170 = local write "I2C_Request"(TRUE ("I2C_Request")) -> ()
                      n171 = Wait (ms)(milliseconds to wait=u32 7) -> ()  [unwired: 1 out]
                    }
                    frame #2 {
                      n172 = local read "Data_Read"() -> (w315:u16)
                      n173 = local write "I2C_Request"(FALSE ("I2C_Request")) -> ()
                      n174 = Equal?(x=w314, y=w315) -> (x = y?=w313:bool)
                      n175 = Equal?(x=w310, y=u16 65535) -> (x = y?=w312:bool)
                      n176 = Or(x=w313, y=w312) -> (x .or. y?=w311:bool)
                      n177 = case shown="False" w311 {
                        tunnel: w317 -> [w323 w334]
                        tunnel: [w324 w334] -> w316
                        tunnel: w310 -> [w322 _]
                        tunnel: w315 -> [w321 _]
                        tunnel: w314 -> [w320 _]
                        frame False {
                          n178 = local read "glitch_num"() -> (w333:i32)
                          n179 = Number To Decimal String(number=w322) -> (decimal integer string=w331:string)  [unwired: 1 in]
                          n180 = Number To Hexadecimal String(2:w321) -> (0:w330:string)  [unwired: 1 in]
                          n181 = Number To Hexadecimal String(2:w320) -> (0:w329:string)  [unwired: 1 in]
                          n182 = Increment(x=w333) -> (x+1=w332:i32)
                          n183 = call <vilib>:"Space Constant.vi"() -> ("String"=w325:string)
                          n184 = local write "glitch_num"(w332) -> ()
                          n185 = Concatenate Strings(w323, "p1#R" ("string"), w331, " rd ", w330, "  df  ", w329, w325) -> (w324:string)
                        }
                        frame True {
                        }
                      }
                      n186 = Wait (ms)(milliseconds to wait=u32 5) -> ()  [unwired: 1 out]
                    }
                  }
                  n187 = Greater Or Equal?(x=w294, y=75) -> (x >= y?=w295:bool)
                  n188 = local read "output enabled"() -> (w299:bool)
                  n189 = local read "IS_SEL"() -> (w298:bool)
                  n190 = Not(x=w299) -> (.not. x?=w297:bool)
                  n191 = Compound Arithmetic op=OR(w295, w297, w298) -> (w296:bool)
                }
                n192 = local write "Glitch Registers"(w288) -> ()
              }
              frame #4 {
                n193 = flat-sequence {
                  frame #0 {
                    n194 = local write "I2C_Write"(TRUE ("I2C_Write")) -> ()
                    n195 = call "I2C_Write.vi"("DataLow"=u8 2 ("Device"), "DataUp"=u8 0 ("Device"), "Reg"=u8 240 ("Device"), "Device"=u8 186) -> ("ArrayLow"=w340:u64, "ArrayUp"=w339:u64)  [unwired: 6 in]
                    n196 = local write "ArrayUp"(w339) -> ()
                    n197 = local write "ArrayLow"(w340) -> ()
                  }
                  frame #1 {
                    n198 = local write "I2C_Request"(TRUE ("I2C_Request")) -> ()
                    n199 = Wait (ms)(milliseconds to wait=u32 5) -> ()  [unwired: 1 out]
                  }
                  frame #2 {
                    n200 = local write "I2C_Request"(FALSE ("I2C_Request")) -> ()
                    n201 = Wait (ms)(milliseconds to wait=u32 5) -> ()  [unwired: 1 out]
                  }
                }
              }
              frame #5 {
                # "PAGE 2"
                n202 = local read "Glitch Registers"() -> (w347:string)
                n203 = local write "I2C_Write"(FALSE ("I2C_Write")) -> ()
                n204 = while {
                  tunnel: "Index - Registers Page 2" -> [w358] mode=indexing
                  tunnel: "Registers Page 2" -> [w361] mode=indexing
                  shift-right: [w359] -> w346
                  shift-left: w347 -> [w360]
                  i -> [w352]
                  stop <- w351 stop-if-true
                  n205 = stacked-sequence {
                    tunnel: w358 -> [w363 _ w368]
                    tunnel: w361 -> [_ _ w372]
                    tunnel: w360 -> [_ _ w375]
                    tunnel: [_ _ w374] -> w359
                    frame #0 {
                      n206 = local write "Device"(u8 186 ("Device")) -> ()
                      n207 = local write "Reg"(w363) -> ()
                      n208 = Wait (ms)(milliseconds to wait=u32 1) -> ()  [unwired: 1 out]
                    }
                    frame #1 {
                      n209 = local write "I2C_Request"(TRUE ("I2C_Request")) -> ()
                      n210 = Wait (ms)(milliseconds to wait=u32 7) -> ()  [unwired: 1 out]
                    }
                    frame #2 {
                      n211 = local read "Data_Read"() -> (w373:u16)
                      n212 = local write "I2C_Request"(FALSE ("I2C_Request")) -> ()
                      n213 = Equal?(x=w372, y=w373) -> (x = y?=w371:bool)
                      n214 = Equal?(x=w368, y=u16 65535) -> (x = y?=w370:bool)
                      n215 = Or(x=w371, y=w370) -> (x .or. y?=w369:bool)
                      n216 = case shown="False" w369 {
                        tunnel: w375 -> [w381 w392]
                        tunnel: [w382 w392] -> w374
                        tunnel: w368 -> [w380 _]
                        tunnel: w373 -> [w379 _]
                        tunnel: w372 -> [w378 _]
                        frame False {
                          n217 = local read "glitch_num"() -> (w391:i32)
                          n218 = Number To Decimal String(number=w380) -> (decimal integer string=w389:string)  [unwired: 1 in]
                          n219 = Number To Hexadecimal String(2:w379) -> (0:w388:string)  [unwired: 1 in]
                          n220 = Number To Hexadecimal String(2:w378) -> (0:w387:string)  [unwired: 1 in]
                          n221 = Increment(x=w391) -> (x+1=w390:i32)
                          n222 = call <vilib>:"Space Constant.vi"() -> ("String"=w383:string)
                          n223 = local write "glitch_num"(w390) -> ()
                          n224 = Concatenate Strings(w381, "p2#R" ("string"), w389, " rd ", w388, "  df  ", w387, w383) -> (w382:string)
                        }
                        frame True {
                        }
                      }
                      n225 = Wait (ms)(milliseconds to wait=u32 5) -> ()  [unwired: 1 out]
                    }
                  }
                  n226 = Greater Or Equal?(x=w352, y=129) -> (x >= y?=w354:bool)
                  n227 = local read "output enabled"() -> (w357:bool)
                  n228 = local read "IS_SEL"() -> (w356:bool)
                  n229 = Not(x=w357) -> (.not. x?=w355:bool)
                  n230 = Compound Arithmetic op=OR(w354, w355, w356) -> (w351:bool)
                }
                n231 = local write "Glitch Registers"(w346) -> ()
              }
              frame #6 {
                w394 = "\r\n"
                w404 = "\t"
                n232 = local read "glitch_num"() -> (w406:i32)
                n233 = local read "glitch_num"() -> (w400:i32)
                n234 = local read "Glitch Registers"() -> (w402:string)
                n235 = local read "Glitch Report"() -> (w395:string)
                n236 = local read "Glitch Registers"() -> (w397:string)
                n237 = Number To Fractional String(number=w406, precision (6)=i16 0 ("width (-)")) -> (F-format string=w405:string)  [unwired: 2 in]
                n238 = Get Date/Time In Seconds() -> (seconds since 1Jan1904=w411:timestamp)
                n239 = Number To Fractional String(number=w400, precision (6)=i16 0 ("width (-)")) -> (F-format string=w398:string)  [unwired: 2 in]
                n240 = Format Date/Time String(time format string (%c)="%d %H:%M:%S:%3u", seconds (now)=w411) -> (date/time string=w413:string)  [unwired: 1 in]
                n241 = Concatenate Strings(w395, "--Report-- ", w398, w394, w397, w394) -> (→"Glitch Report":string)
                n242 = local read "GLITCH_log file"() -> (w410:refnum<file>)
                n243 = Concatenate Strings(w413, w404, w405, w404, w402, "\r\n") -> (w412:string)
                n244 = Format Into String(initial string=w410, w412) -> (resulting string=w409:refnum<file>)  [unwired: 2 in, 1 out]
                n245 = local write "GLITCH_log file"(w409) -> ()
              }
            }
          }
        }
        n246 = local write "Comand"(w152) -> ()
      }
    }
    n247 = local read "stop"() -> (w151:bool)
    n248 = Wait (ms)(milliseconds to wait=u32 1) -> ()  [unwired: 1 out]
  }
  n249 = while {
    tunnel: w2 -> [_]
    stop <- w415 stop-if-true
    # "Парирование тиристора"
    n250 = stacked-sequence {
      frame #0 {
        n251 = local read "VDDIO_Current, mA"() -> (w423:dbl)
        n252 = local read "VAA_Current, mA"() -> (w424:dbl)
        n253 = local read "VDD_Current, mA"() -> (w428:dbl)
        n254 = Greater Or Equal?(x=w424, y="VAA_limit, mA") -> (x >= y?=w420:bool)
        n255 = Greater Or Equal?(x=w428, y="VDD_limit, mA") -> (x >= y?=w418:bool)
        n256 = Greater Or Equal?(x=w423, y="VDDIO_limit, mA") -> (x >= y?=w422:bool)
        n257 = case shown="True" w420 {
          tunnel: [FALSE TRUE] -> w419
          frame False {
          }
          frame True {
            n258 = local read "selNumVAA"() -> (w436:i32)
            n259 = Increment(x=w436) -> (x+1=w435:i32)
            n260 = local write "selNumVAA"(w435) -> ()
          }
        }
        n261 = case shown="True" w418 {
          tunnel: [FALSE TRUE] -> w417
          frame False {
          }
          frame True {
            n262 = local read "selNumVDDIO"() -> (w432:i32)
            n263 = Increment(x=w432) -> (x+1=w431:i32)
            n264 = local write "selNumVDDIO"(w431) -> ()
          }
        }
        n265 = case shown="True" w422 {
          tunnel: [FALSE TRUE] -> w421
          frame False {
          }
          frame True {
            n266 = local read "selNumVDD"() -> (w440:i32)
            n267 = Increment(x=w440) -> (x+1=w439:i32)
            n268 = local write "selNumVDD"(w439) -> ()
          }
        }
        n269 = Compound Arithmetic op=OR(w421, w419, w417) -> (→"IS_SEL":bool)
      }
      frame #1 {
        n270 = case shown="True" "WRITE\nSEL_LOG" {
          frame False {
          }
          frame True {
            w448 = i16 0 ("width (-)")
            w447 = i16 3 ("width (-)")
            w445 = "\t"
            n271 = local read "VAA_Current, mA"() -> (w462:dbl)
            n272 = local read "VDDIO_Current, mA"() -> (w460:dbl)
            n273 = local read "VDD_Current, mA"() -> (w461:dbl)
            n274 = local read "selNumVDDIO"() -> (w463:i32)
            n275 = local read "selNumVDD"() -> (w464:i32)
            n276 = local read "selNumVAA"() -> (w465:i32)
            n277 = local read "SIM_SEL"() -> (w452:bool)
            n278 = local read "IS_SEL"() -> (w453:bool)
            n279 = Compound Arithmetic op=OR(w453, w452) -> (w469:bool)
            n280 = Number To Fractional String(number=w460, precision (6)=w447) -> (F-format string=w466:string)  [unwired: 2 in]
            n281 = Number To Fractional String(number=w461, precision (6)=w447) -> (F-format string=w467:string)  [unwired: 2 in]
            n282 = Number To Fractional String(number=w462, precision (6)=w447) -> (F-format string=w468:string)  [unwired: 2 in]
            n283 = Number To Fractional String(number=w463, precision (6)=w448) -> (F-format string=w456:string)  [unwired: 2 in]
            n284 = Number To Fractional String(number=w464, precision (6)=w448) -> (F-format string=w455:string)  [unwired: 2 in]
            n285 = Number To Fractional String(number=w465, precision (6)=w448) -> (F-format string=w454:string)  [unwired: 2 in]
            n286 = Select(t="!!SEL!!", s=w469, f=" ") -> (s? t:f=w451:string)
            n287 = Get Date/Time In Seconds() -> (seconds since 1Jan1904=w457:timestamp)
            n288 = Format Date/Time String(time format string (%c)="%d %H:%M:%S:%3u", seconds (now)=w457) -> (date/time string=w459:string)  [unwired: 1 in]
            n289 = local read "SEL_log file"() -> (w443:refnum<file>)
            n290 = Concatenate Strings(w459, w445, w466, w445, w467, w445, w468, w445, w456, w445, w455, w445, w454, w445, w451, "\r\n") -> (w458:string)
            n291 = Format Into String(initial string=w443, w458) -> (resulting string=w442:refnum<file>)  [unwired: 2 in, 1 out]
            n292 = local write "SEL_log file"(w442) -> ()
          }
        }
      }
      frame #2 {
        n293 = local read "IS_SEL"() -> (w470:bool)
        n294 = case shown="True" w470 {
          frame False {
          }
          frame True {
            n295 = flat-sequence {
              frame #0 {
                n296 = local write "INIT_REGISTERS"(FALSE ("INIT_REGISTERS")) -> ()
                n297 = local write "output enabled"(FALSE ("output enabled")) -> ()
                n298 = Wait (ms)(milliseconds to wait="SEL_time") -> ()  [unwired: 1 out]
              }
              frame #1 {
                n299 = local write "output enabled"(TRUE ("output enabled")) -> ()
                n300 = Wait (ms)(milliseconds to wait=u32 2) -> ()  [unwired: 1 out]
              }
              frame #2 {
                n301 = local write "INIT_REGISTERS"(TRUE ("INIT_REGISTERS")) -> ()
                n302 = local write "IS_SEL"(FALSE ("IS_SEL")) -> ()
              }
            }
          }
        }
      }
    }
    n303 = local read "stop"() -> (w415:bool)
    n304 = Wait (ms)(milliseconds to wait=u32 300) -> ()  [unwired: 1 out]
  }
  n305 = while {
    tunnel: w7 -> [w494]
    tunnel: [w493] -> w9
    tunnel: w4 -> [w480]
    tunnel: [w481] -> w3
    stop <- w495 stop-if-true
    w484 = T5 0 items=["Current", "Voltage"] ("measurement type")
    w485 = T5 1 items=["Current", "Voltage"] ("measurement type")
    # "Управление источниками"
    n306 = stacked-sequence {
      tunnel: w494 -> [w506 w511]
      tunnel: [_ w510] -> w493
      tunnel: "output enabled" -> [w496 w512]
      frame #0 {
        w499 = T5 0 items=["Current", "Voltage"] ("measurement type")
        w500 = T5 1 items=["Current", "Voltage"] ("measurement type")
        n307 = call <instrlib>:"niDCPower Configure Output Enabled.vi"("output enabled"=w496, "channel name"="1", "instrument handle"=w506) -> ("instrument handle out"=w508:refnum<k15>)  [unwired: 7 in, 1 out]
        n308 = call <instrlib>:"niDCPower Measure.vi"("measurement type"=w500, "channel name"="1", "instrument handle"=w508) -> ("measurement"=→"VDD_Voltage, V":dbl, "instrument handle out"=w505:refnum<k15>)  [unwired: 6 in, 1 out]
        n309 = call <instrlib>:"niDCPower Measure.vi"("measurement type"=w499, "channel name"="1", "instrument handle"=w505) -> ("measurement"=w501:dbl)  [unwired: 6 in, 2 out]
        n310 = Multiply(x=w501, y=1000.0) -> (x*y=→"VDD_Current, mA":dbl)
      }
      frame #1 {
        w517 = T5 0 items=["Current", "Voltage"] ("measurement type")
        w515 = T5 1 items=["Current", "Voltage"] ("measurement type")
        n311 = call <instrlib>:"niDCPower Configure Output Enabled.vi"("output enabled"=w512, "channel name"="0", "instrument handle"=w511) -> ("instrument handle out"=w519:refnum<k15>)  [unwired: 7 in, 1 out]
        n312 = call <instrlib>:"niDCPower Measure.vi"("measurement type"=w515, "channel name"="0", "instrument handle"=w519) -> ("measurement"=→"VDDIO_Voltage, V":dbl, "instrument handle out"=w520:refnum<k15>)  [unwired: 6 in, 1 out]
        n313 = call <instrlib>:"niDCPower Measure.vi"("measurement type"=w517, "channel name"="0", "instrument handle"=w520) -> ("measurement"=w521:dbl, "instrument handle out"=w510:refnum<k15>)  [unwired: 6 in, 1 out]
        n314 = Multiply(x=w521, y=1000.0) -> (x*y=→"VDDIO_Current, mA":dbl)
      }
    }
    n315 = call <instrlib>:"niDCPower Configure Output Enabled.vi"("output enabled"="output enabled", "channel name"="0", "instrument handle"=w480) -> ("instrument handle out"=w492:refnum<k15>)  [unwired: 7 in, 1 out]
    n316 = call <instrlib>:"niDCPower Measure.vi"("measurement type"=w485, "channel name"="0", "instrument handle"=w492) -> ("measurement"=→"VAA_Voltage, V":dbl, "instrument handle out"=w490:refnum<k15>)  [unwired: 6 in, 1 out]
    n317 = call <instrlib>:"niDCPower Measure.vi"("measurement type"=w484, "channel name"="0", "instrument handle"=w490) -> ("measurement"=w486:dbl, "instrument handle out"=w481:refnum<k15>)  [unwired: 6 in, 1 out]
    n318 = Multiply(x=w486, y=1000.0) -> (x*y=→"VAA_Current, mA":dbl)
    n319 = local read "stop"() -> (w495:bool)
    n320 = Wait (ms)(milliseconds to wait=u32 1) -> ()  [unwired: 1 out]
  }
  n321 = while {
    shift-right: ["INIT_REGISTERS"] -> _
    shift-left: FALSE -> [w526]
    tunnel: w2 -> [_]
    stop <- w527 stop-if-true
    # "Инициализация"
    n322 = Greater?(x="INIT_REGISTERS", y=w526) -> (0:w525:bool)
    n323 = case shown="True" w525 {
      frame False {
      }
      frame True {
        n324 = stacked-sequence {
          frame #0 {
            n325 = local write "/RESET"(FALSE ("RESET")) -> ()
            n326 = Wait (ms)(milliseconds to wait=u32 50) -> ()  [unwired: 1 out]
          }
          frame #1 {
            n327 = local write "/RESET"(TRUE ("RESET")) -> ()
            n328 = Wait (ms)(milliseconds to wait=u32 20) -> ()  [unwired: 1 out]
          }
          frame #2 {
            n329 = flat-sequence {
              frame #0 {
                n330 = local write "Comand"(T1."250x250" ("Comand")) -> ()
              }
              frame #1 {
                n331 = local write "Comand"(TRUE) -> ()
                n332 = Wait (ms)(milliseconds to wait=u32 50) -> ()  [unwired: 1 out]
              }
            }
          }
          frame #3 {
            n333 = flat-sequence {
              frame #0 {
                n334 = local write "Comand"(T1."RGB565" ("Comand")) -> ()
              }
              frame #1 {
                n335 = Wait (ms)(milliseconds to wait=u32 50) -> ()  [unwired: 1 out]
                n336 = local write "Comand"(TRUE) -> ()
              }
            }
            n337 = local write "INIT_REGISTERS"(FALSE) -> ()
          }
        }
      }
    }
    n338 = local read "stop"() -> (w527:bool)
    n339 = Wait (ms)(milliseconds to wait=u32 1) -> ()  [unwired: 1 out]
  }
  n340 = while {
    tunnel: w2 -> [_]
    stop <- w544 stop-if-true
    n341 = local read "output enabled"() -> (w542:bool)
    n342 = local read "REGISTERS"() -> (w541:bool)
    n343 = local read "IS_SEL"() -> (w540:bool)
    n344 = Not(x=w540) -> (.not. x?=w539:bool)
    n345 = Compound Arithmetic op=AND(w541, w542, w539) -> (w543:bool)
    n346 = case shown="True" w543 {
      frame False {
      }
      frame True {
        n347 = flat-sequence {
          frame #0 {
            n348 = local write "Comand"(T1."check_registers" ("Comand")) -> ()
          }
          frame #1 {
            n349 = local write "Comand"(TRUE) -> ()
            n350 = Wait (ms)(milliseconds to wait=u32 100) -> ()  [unwired: 1 out]
          }
        }
      }
    }
    n351 = local read "stop"() -> (w544:bool)
  }
  n352 = while {
    tunnel: w5 -> [_]
    stop <- w550 stop-if-true
    # "Преобразование данных в картинку IMAQ для VISION"
    n353 = local read "Ready"() -> (w548:bool)
    n354 = case shown="True" w548 {
      frame False {
      }
      frame True {
        w557 = T6 4 items=["Grayscale (U8)", "Grayscale (I16)", "Grayscale (SGL)", "Complex (CSG)", "RGB (U32)", "HSL (U32)", "RGB (U64)"] ("Image Type")
        n355 = local read "Data"() -> (w552:u8[])
        n356 = for {
          N: "Height_pix" -> [_]
          shift-right: [w564] -> _
          shift-left: w552 -> [w561]
          tunnel: [w562] -> w553 mode=indexing
          w566 = u16 0 items=["RGB", "HSL", "HSV", "HSI"] ("Color Mode")
          # "RGB565"
          n357 = Multiply(x="Width_pix", y=2) -> (x*y=w560:i32)
          n358 = Split 1D Array(array=w561, index=w560) -> (second subarray=w564:u8[])  [unwired: 1 out]
          n359 = Decimate 1D Array(w564) -> (w568:u8[], w567:u8[])
          n360 = for {
            N: "Width_pix" -> [_]
            tunnel: w568 -> [w587] mode=indexing
            tunnel: w567 -> [w588] mode=indexing
            tunnel: [w569] -> w563 mode=indexing
            w577 = FALSE
            w578 = FALSE
            w579 = FALSE
            # "BLUE"
            # "GREEN"
            # "RED"
            # "SECOND"
            # "FIRST"
            n361 = Number To Boolean Array(number=w588) -> (Boolean array=w583:bool[])
            n362 = Number To Boolean Array(number=w587) -> (Boolean array=w586:bool[])
            n363 = Split 1D Array(array=w583, index=5) -> (first subarray=w575:bool[], second subarray=w582:bool[])
            n364 = Split 1D Array(array=w586, index=3) -> (first subarray=w574:bool[], second subarray=w573:bool[])
            n365 = Build Array (concatenate)(w578, w578, w582, w574) -> (w581:bool[])
            n366 = Build Array (concatenate)(w579, w579, w579, w573) -> (w580:bool[])
            n367 = Boolean Array To Number(Boolean array=w581) -> (number=w571:u8)
            n368 = Boolean Array To Number(Boolean array=w580) -> (number=w570:u8)
            n369 = Build Array (concatenate)(w577, w577, w577, w575) -> (w576:bool[])
            n370 = Boolean Array To Number(Boolean array=w576) -> (number=w572:u8)
            n371 = Bundle(w570, w571, w572) -> (w569:cluster{u8, u8, u8})  [unwired: 1 in]
          }
          n372 = call "IMAQ ColorValueToInteger"("1D Color value array"=w563, "Color Mode"=w566) -> ("1D U32 array"=w562:u32[])  [unwired: 3 in, 3 out]
        }
        n373 = call "IMAQ Create"("Image Name"="Kek", "Image Type"=w557) -> ("New Image"=w556:T2)  [unwired: 3 in, 1 out]
        n374 = local write "Ready"(FALSE ("Ready")) -> ()
        n375 = call "IMAQ ArrayToColorImage"("Image Pixels (U32)"=w553, "Image"=w556) -> ("Image Out"=→"Image":T2)  [unwired: 3 in, 1 out]
      }
    }
    n376 = local read "stop"() -> (w550:bool)
    n377 = Wait (ms)(milliseconds to wait=u32 10) -> ()  [unwired: 1 out]
  }
  n378 = while {
    tunnel: w2 -> [w648]
    tunnel: [w648] -> w12
    shift-right: [w630] -> _
    shift-left: FALSE -> [w649]
    tunnel: w5 -> [_]
    shift-right: [w611] -> _
    shift-left: TRUE -> [w612]
    stop <- w610 stop-if-true
    # "Массивы переворачиваются!!!!!!"
    n379 = local read "Device"() -> (w607:u8)
    n380 = local read "ArrayLow"() -> (w624:u64)
    n381 = local read "ArrayUp"() -> (w623:u64)
    n382 = Increment(x=w607) -> (x+1=w606:u8)
    n383 = local read "Reg"() -> (w605:u8)
    n384 = xnode "Read/Write Control"("FPGA VI Reference In"=w648, "I2C_Write"="I2C_Write", "Read2"="Read2", "Read1"="Read1", "Device_Read"=w606, "Reg"=w605, "Device_Write"=w607, "91"="91", "100_Sclk_divider"="100_Sclk_divider", "75_Stop"="75_Stop", "53"="53", "35"="35", "17"="17", "71"="71", "54"="54", "36"="36", "18"="18", "72"="72", "50_Rise/Fall divider"="50_Rise/Fall divider", "0_WE divider"="0_WE divider", "DataUp"=w623, "DataLow"=w624, "I2C_Request"="I2C_Request", "FALSE_LV"="FALSE_LV", "FALSE_PIXCLK"="FALSE_PIXCLK", "TRUE_FV"="TRUE_FV", "Остановите"="stop", "Читай_Линию"=w612, "1_EXTCLK_divider"="1_EXTCLK_divider", "String_number"="String_number", "55"="55", "56"="56", "75"="75", "73"="73", "55"="55", "RESET"="/RESET", "57"="57") -> ("FPGA VI Reference Out"=w647:refnum<k20>, "Линия_готова_на_все"=w630:bool, "ACK"=w619:bool[], "String_counter"=→"String_counter":i16, "READ_Number"=w591:u64)  [unwired: 2 in, 3 out]
    "number" <- w591
    n385 = Number To Boolean Array(number=w591) -> (Boolean array=w592:bool[])
    n386 = Greater?(x=w630, y=w649) -> (0:w620:bool)
    n387 = Boolean Array To Number(Boolean array=w619) -> (number=→"ACK":u8)
    n388 = case shown="True" w620 {
      tunnel: w647 -> [_ w677]
      tunnel: [TRUE FALSE ("Читай_Линию")] -> w611
      frame False {
      }
      frame True {
        # "Чтение из FIFO данных (картинка)"
        n389 = xnode "Invoke Method"("FPGA VI Reference In"=w677, "Number of Elements"=u32 0, "Timeout (ms)"=0) -> ("FPGA VI Reference Out"=w682:refnum<k20>, "error out"=w681:errorcluster, "Elements Remaining"=w673:u32)  [unwired: 1 in, 1 out]
        "Сколько вначале" <- w673
        n390 = xnode "Invoke Method"("FPGA VI Reference In"=w682, "error in"=w681, "Number of Elements"=w673, "Timeout (ms)"=0) -> ("FPGA VI Reference Out"=w674:refnum<k20>, "Data"=→"Data":u8[])  [unwired: 2 out]
        n391 = Not(x=TRUE) -> (.not. x?=w675:bool)
        n392 = xnode "Read/Write Control"("FPGA VI Reference In"=w674, "Линия_ прочтена"=w675) -> ()  [unwired: 1 in, 2 out]
        "Ready" <- TRUE ("Ready")
      }
    }
    n393 = Split 1D Array(array=w592, index=6) -> (second subarray=w603:bool[])  [unwired: 1 out]
    n394 = Split 1D Array(array=w603, index=16) -> (first subarray=w601:bool[], second subarray=w599:bool[])
    n395 = for {
      tunnel: w601 -> [w660] mode=indexing
      shift-right: [w659] -> w600
      shift-left: bool[] [] -> [w658]
      tunnel: w599 -> [w652] mode=indexing
      shift-right: [w651] -> w598
      shift-left: bool[] [] -> [w650]
      i -> [w655]
      n396 = Quotient & Remainder(x=w655, y=2) -> (x-y*floor(x/y)=w657:i32)  [unwired: 1 out]
      n397 = Equal?(x=w657, y=1) -> (x = y?=w656:bool)
      n398 = case shown="True" w656 {
        tunnel: w660 -> [_ w668]
        tunnel: [w662 w667] -> w659
        tunnel: w658 -> [w662 w666]
        tunnel: w652 -> [_ w665]
        tunnel: [w661 w664] -> w651
        tunnel: w650 -> [w661 w663]
        frame False {
        }
        frame True {
          n399 = Build Array (concatenate)(w668, w666) -> (w667:bool[])
          n400 = Build Array (concatenate)(w665, w663) -> (w664:bool[])
        }
      }
    }
    n401 = Boolean Array To Number(Boolean array=w600) -> (number=w590:u8)
    "Read_Up" <- w590
    n402 = Boolean Array To Number(Boolean array=w598) -> (number=w589:u8)
    "Read_Low" <- w589
    n403 = Join Numbers(hi=w590, lo=w589) -> ((hi.lo)=→"Data_Read":u16)
    n404 = local read "stop"() -> (w610:bool)
    n405 = Wait (ms)(milliseconds to wait=u32 1) -> ()  [unwired: 1 out]
  }
  n406 = flat-sequence {
    tunnel: w9 -> [w685]
    frame #0 {
      n407 = call <instrlib>:"niDCPower Configure Output Enabled.vi"("output enabled"=FALSE, "instrument handle"=w685) -> ("instrument handle out"=w683:refnum<k15>)  [unwired: 8 in, 1 out]
      n408 = call <instrlib>:"niDCPower Close.vi"("instrument handle"=w683) -> ()  [unwired: 10 in, 1 out]
    }
  }
  n409 = flat-sequence {
    tunnel: w3 -> [w688]
    frame #0 {
      n410 = call <instrlib>:"niDCPower Configure Output Enabled.vi"("output enabled"=FALSE, "instrument handle"=w688) -> ("instrument handle out"=w686:refnum<k15>)  [unwired: 8 in, 1 out]
      n411 = call <instrlib>:"niDCPower Close.vi"("instrument handle"=w686) -> ()  [unwired: 10 in, 1 out]
    }
  }
  n412 = xnode "Close FPGA VI Reference"("FPGA VI Reference In"=w12) -> ()  [unwired: 1 in, 1 out]
